vi "SwissSPAD Live_Filter Error.vi"(8 "error in (no error)":errorcluster, 11 "SS2 Q Elements in":T1[](array[typedef])) -> (0 "error out":errorcluster, 3 "SS2 Q Elements out":T1[](array[typedef]))   [LabVIEW 2021]
uses:
  SwissSPAD Live_Q [Element].ctl
  SwissSPAD Live_Q Event List.ctl
  SwissSPAD Live_Settings List.ctl
  SwissSPAD Live_Internal Data List.ctl
  Variant/Variant to Data/Variant to Data.lvlib
  Notebook/Notebook.lvlib
  Rich Text Box/Rich Text Box.lvlib
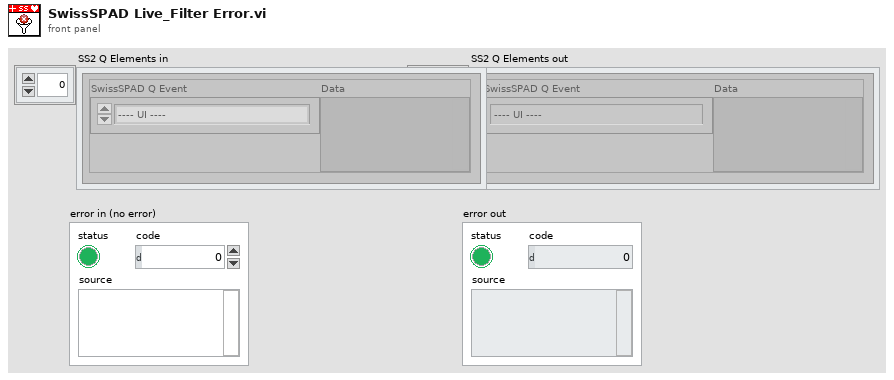
[diagram p1: front panel]
types:
  T1 = typedef "SwissSPAD Live_Q [Element].ctl" = cluster{"SwissSPAD Q Event":T2, "Data":variant}
  T2 = typedef "SwissSPAD Live_Q Event List.ctl" = enum16{"---- UI ----", "Idle", "Initialization", "Init FPGA(s)", "Init Top FPGA (deprecated)", "FPGA(s) Status", "Top FPGA Status (deprecated)", "Reset FPGA(s)", "Reset Top FPGA (deprecated)", "Refresh Display Image", "Quit", "---- DAQ ----", "Start Recording", "Start Live Acquisition", "Initialize Recording Mode", "Initialize FPGA (Live Mode)", "Get Image Set", "Get Single Image", "Update Image Display", "Stop Live Acquisition", "Stop Data Recording", "Stop Data Saving", "---- Image ----", "Copy Data to Clipboard", "Set Image Palette", "Save Displayed Image with Overlay", "Save Image Data as TIFF"}
  T3 = typedef "SwissSPAD Live_Settings List.ctl" = enum16{"FPGA:Bottom Half", "FPGA:Top Half", "FPGA:Bottom Bitfile Path", "FPGA:Top Bitfile Path", "FPGA:Bottom Bitstream Version", "FPGA:Top Bitstream Version", "FPGA:Auto Reset FPGA", "FPGA:Bottom FPGA Serial Number", "FPGA:Top FPGA Serial Number", "FPGA:Detector PCB Version", "Acquisition Parameters:Microlens", "Acquisition Parameters:SS2 DAQ Parameters", "Acquisition Parameters:Gate Configuration Array", "Acquisition Parameters:SS3 DAQ Parameters", "Acquisition Parameters:Buffer Size (# 8-bit Gates)", "File Information:File Information", "File Information:# Datasets in Series", "File Information:Scrambled File Flag", "File Information:SS3 Gate Slip Correction", "File Information:SS3 Hot Pixel Mismatch Detection", "File Information:Delay between Datasets", "File Information:Save Sum of All Gates Preview", "Image Parameters:Image ROI Information", "Image Parameters:Image Binning Options", "Image Parameters:SS3 Displayed Image", "Image Parameters:Image Display Options", "Image Parameters:Use Histogram Cursors", "Image Parameter:FPGA Data to Display", "UI Settings:Histogram Bins Number", "UI Settings:Use Image Display Options", "UI Settings:Verbose Settings", "UI Settings:Verbose Saving"}
  T4 = typedef "SwissSPAD Live_Internal Data List.ctl" = enum16{"Number of pending file saving tasks", "File Saving Tasks Information", "Current Image ROI Information", "# FPGA Reset Attempts", "Histogram Cursor Locations", "Histogram Window is Open"}
  T5 = typedef "Rich Text Box.lvlib/Text Formatting.ctl" = cluster{"Font":string, "Text Color":T6, "Text Background Color":T6, "Text Style":enum16{"Regular", "Bold", "Italic", "Underline", "Strikeout"}, "Font Size (Points)":dbl, "Text Alignment":i32}
  T6 = typedef "Rich Text Box.lvlib/Text Colors.ctl" = enum16{"Unchanged", "Black", "Blue", "Brown", "Gray", "Green", "Orange", "Pink", "Red", "White"}
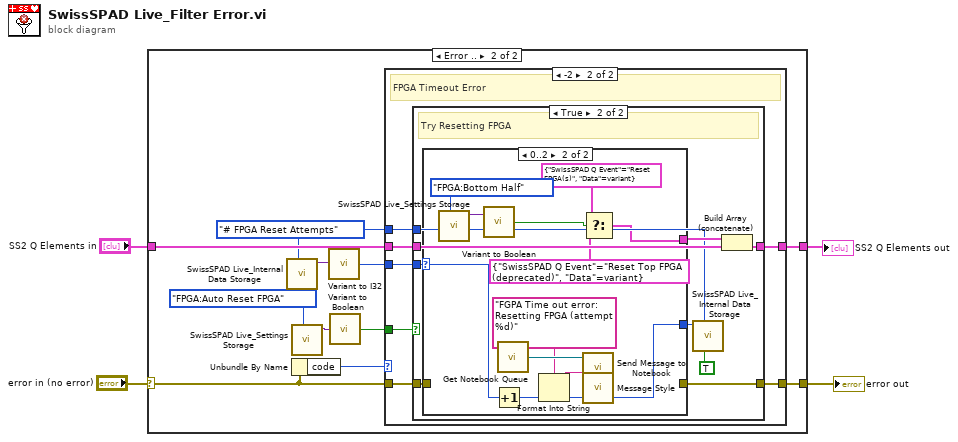
[diagram p0: block diagram]
diagram:
  n1 = case shown="Error .." "error in (no error)" {
    selector: "error in (no error)" -> [w5 w16]
    tunnel: "SS2 Q Elements in" -> [w6 w14]
    tunnel: [w6 w12] -> w2
    tunnel: [w5 w15] -> w1
    frame No Error {
    }
    frame Error {
      w9 = SwissSPAD_Live_Internal_Data_List."# FPGA Reset Attempts" ("SS2 Live Data")
      n2 = call "SwissSPAD Live_Internal Data Storage.vi"("SS2 Live Data"=w9) -> ("Variant"=w11:variant)  [unwired: 8 in, 2 out]
      n3 = call "SwissSPAD Live_Settings Storage.vi"("Settings List"=SwissSPAD_Live_Settings_List."FPGA:Auto Reset FPGA") -> ("Variant Data out"=w7:variant)  [unwired: 9 in, 1 out]
      n4 = Unbundle By Name(w16) -> ("code"=w17:i32)
      n5 = call "Variant to I32.vi"("Variant"=w11) -> ("Value"=w10:i32)  [unwired: 8 in]
      n6 = call "Variant to Boolean.vi"("Variant"=w7) -> ("Value"=w13:bool)  [unwired: 8 in]
      n7 = case shown="-2" w17 {
        tunnel: w16 -> [w19 w23]
        tunnel: [w19 w22] -> w15
        tunnel: w14 -> [w18 w25]
        tunnel: w13 -> [_ w26]
        tunnel: [w18 w24] -> w12
        tunnel: w10 -> [_ w21]
        tunnel: w9 -> [_ w20]
        frame 0, Default {
        }
        frame -2 {
          # "FPGA Timeout Error"
          n8 = case shown="True" w26 {
            tunnel: w25 -> [w28 w37]
            tunnel: [w28 w36] -> w24
            tunnel: w23 -> [w27 w34]
            tunnel: [w27 w33] -> w22
            tunnel: w21 -> [_ w32]
            tunnel: w20 -> [_ w30]
            frame False {
            }
            frame True {
              # "Try Resetting FPGA"
              n9 = case shown="0..2" w32 {
                selector: w32 -> [_ w46]
                tunnel: [_ w41] -> w35
                tunnel: w34 -> [w38 _]
                tunnel: [w38 _] -> w33
                tunnel: [_ w45] -> w29
                frame 3, Default {
                  # "Don't reset if 3 attempts have been made"
                }
                frame 0..2 {
                  n10 = call "SwissSPAD Live_Settings Storage.vi"("Settings List"=SwissSPAD_Live_Settings_List."FPGA:Bottom Half") -> ("Variant Data out"=w39:variant)  [unwired: 9 in, 1 out]
                  n11 = call "Variant to Boolean.vi"("Variant"=w39) -> ("Value"=w44:bool)  [unwired: 8 in]
                  n12 = Increment(x=w46) -> (x+1=w45:i32)
                  n13 = call "Get Notebook Queue.vi"() -> ("Notebook Queue"=w49:refnum<queue>)  [unwired: 9 in]
                  n14 = Format Into String(format string="FGPA Time out error: Resetting FPGA (attempt %d)" ("Message"), w45) -> (resulting string=w47:string)  [unwired: 2 in, 1 out]
                  n15 = call "Message Style.vi"() -> ("Message Formatting"=w50:T5)
                  n16 = call "Send Message to Notebook.vi"("Text Formatting"=w50, "Message"=w47, "Notebook Queue"=w49) -> ()  [unwired: 5 in, 2 out]
                  n17 = Select(t=T1 {"SwissSPAD Q Event"=enum."Reset FPGA(s)", "Data"=variant} ("element"), s=w44, f=T1 {"SwissSPAD Q Event"=enum."Reset Top FPGA (deprecated)", "Data"=variant} ("element")) -> (s? t:f=w41:T1)
                }
              }
              n18 = call "SwissSPAD Live_Internal Data Storage.vi"("Get(F)/Set"=TRUE, "SS2 Live Data"=w30, "Variant"=w29) -> ()  [unwired: 6 in, 3 out]
              n19 = Build Array (concatenate)(w35, w37) -> (w36:T1[])
            }
          }
        }
      }
    }
  }
  "error out" <- w1
  "SS2 Q Elements out" <- w2
